vi "DAQ_AI_acquire.vi"(3 "Error In":errorcluster, 5 "DAQmx Task Name":refnum<k21>) -> (0 "Error Out":errorcluster, 1 "data":dbl[][](array[numeric]) format="%0.2f", 2 "task out":refnum<k21>)   [LabVIEW 2020]
uses:
  <vilib>/DAQmx/read.llb/DAQmx Read (Analog 2D DBL NChan NSamp).vi
  <vilib>/DAQmx/miscellaneous.llb/DAQmx Fill In Error Info.vi
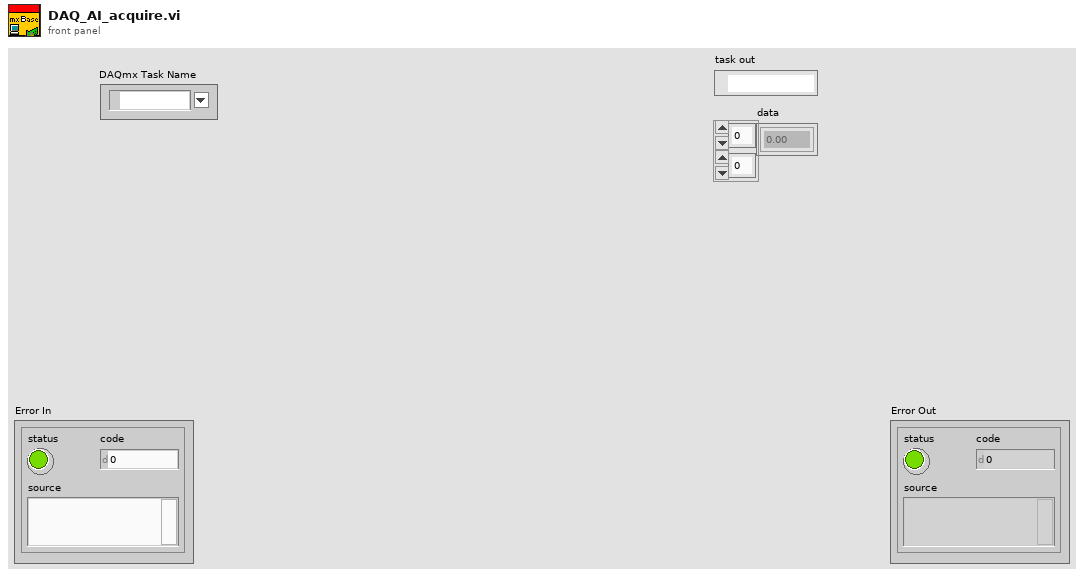
[diagram p1: front panel]
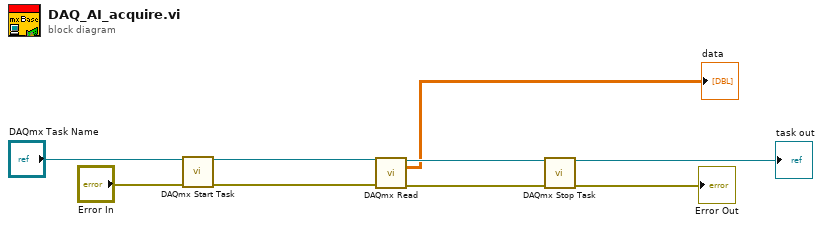
[diagram p0: block diagram]
diagram:
  n1 = call <vilib>:"DAQmx Start Task.vi"("task/channels in"="DAQmx Task Name", "error in"="Error In") -> ("task out"=w6:refnum<k21>, "error out"=w7:errorcluster)  [unwired: 12 in]
  n2 = call-poly <vilib>:"DAQmx Read.vi"("task/channels in"=w6, "error in"=w7) -> ("task out"=w5:refnum<k21>, "data"=→"data":dbl[][], "error out"=w4:errorcluster)  [unwired: 11 in]
  n3 = call <vilib>:"DAQmx Stop Task.vi"("task/channels in"=w5, "error in"=w4) -> ("task out"=→"task out":refnum<k21>, "error out"=→"Error Out":errorcluster)  [unwired: 12 in]
